vi "Custom Aggregation (Complex Spectra).vi"(0 "complex spectra":cluster{"f0":dbl, "df":dbl, "vectors":cdb[]}[](array[cluster]), 1 "reset? (F)":bool, 5 "aggregation settings":T1={"interval"=1, "interval unit"=enum."Runs", "synchronization of intervals"=enum."Not synchronized", "algorithm"=enum."Average"}, 9 "system info in":refnum<class "EP System Info.lvclass">, 11 "error in (no error)":errorcluster, 12 "data timestamp":timestamp) -> (4 "aggregated minimum values":T2(array[cluster]), 6 "aggregated averaged/RMS values":T2(array[cluster]), 8 "aggregated maximum values":T2(array[cluster]), 10 "system info out":refnum<class "EP System Info.lvclass">, 13 "aggregated data valid?":bool, 14 "aggregated data timestamp":timestamp, 15 "error out":errorcluster)   [LabVIEW 2014, in "NI_EP_Power Quality.lvlib"]
doc: "Calculates the aggregated minimum, maximum, and averaged or RMS value of an input signal for a specified aggregation interval, according to Class S in IEC 61000-4-30:2008. There is no overlap between aggregation intervals. This VI automatically restarts accumulation at the beginning of the next time interval after the previous interval expires. You must manually select the polymorphic instance you want to use.\n\nThis VI supports measuring single-line and multiple-line systems except the DBL instance. Use the DBL instance to measure one channel on one line at one time."
uses:
  <vilib>/addons/Electrical Power/PQ/NI_EP_Power Quality.lvlib
  <vilib>/addons/Electrical Power/PQ/Common/Controls/ep_Aggregation Settings.ctl
  <vilib>/addons/Electrical Power/PQ/Common/Classes/System Info/EP System Info.lvclass
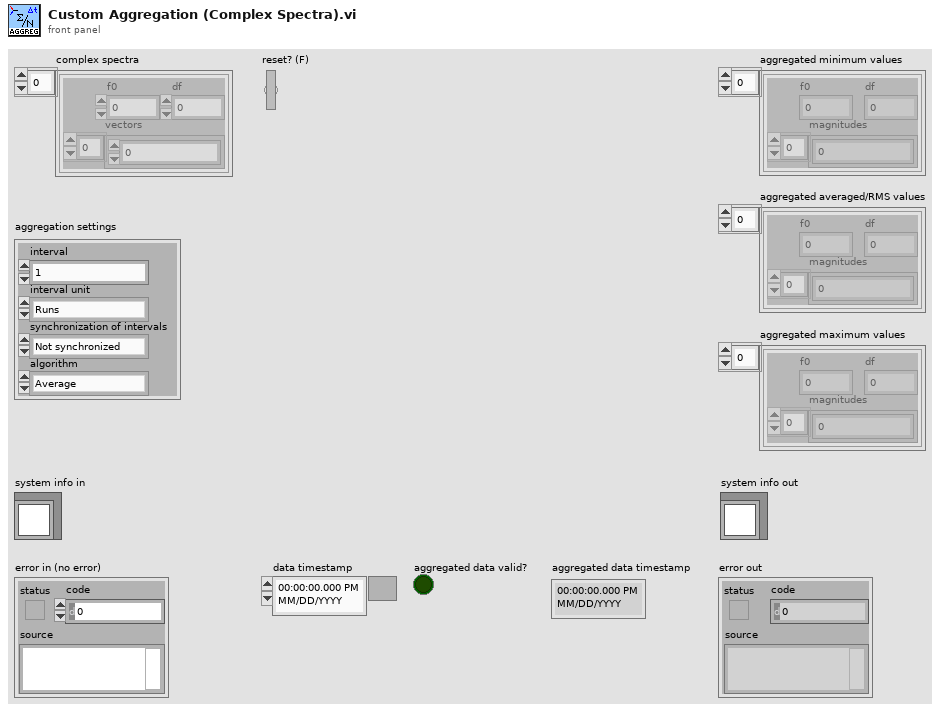
[diagram p1: front panel]
types:
  T1 = typedef "NI_EP_Power Quality.lvlib/ep_Aggregation Settings.ctl" = cluster{"interval":u32, "interval unit":enum16{"Runs", "Seconds", "Minutes", "Hours", "Days", "Weeks"}, "synchronization of intervals":enum16{"Not synchronized", "Interval rounded"}, "algorithm":enum16{"Average", "RMS"}}
  T2 = cluster{"f0":dbl, "df":dbl, "magnitudes":dbl[]}[]
  T3 = cluster{"f0":dbl, "df":dbl, "amplitudes":dbl[]}[]
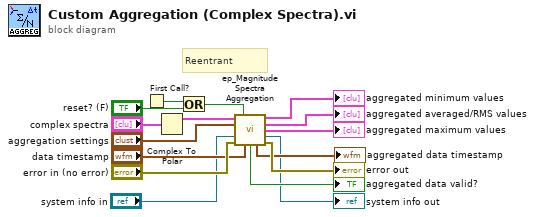
[diagram p0: block diagram]
diagram:
  # "Reentrant"
  n1 = First Call?() -> (First Call?: T/F=w8:bool)
  n2 = Complex To Polar(r * e^(i*theta)="complex spectra") -> (r=w13:cluster{"f0":dbl, "df":dbl, "vectors":dbl[]}[])  [unwired: 1 out]
  n3 = Or(x=w8, y="reset? (F)") -> (x .or. y?=w6:bool)
  n4 = call <vilib>:"ep_Magnitude Spectra Aggregation.vi"("spectra"=w13, "reset? (F)"=w6, "aggregation settings"="aggregation settings", "system info in"="system info in", "error in (no error)"="error in (no error)", "data timestamp"="data timestamp") -> ("aggregated minimum values"=→"aggregated minimum values":T3, "aggregated avgeraged/RMS values"=→"aggregated averaged/RMS values":T3, "aggregated maximum values"=→"aggregated maximum values":T3, "system info out"=→"system info out":refnum<class "EP System Info.lvclass">, "aggregated data valid?"=→"aggregated data valid?":bool, "aggregated data timestamp"=→"aggregated data timestamp":timestamp, "error out"=→"error out":errorcluster)  [unwired: 3 in]
